vi "통신.vi"(8 "error in":errorcluster) -> (0 "error out":errorcluster, 3 "Boolean":bool)   [LabVIEW 2023]
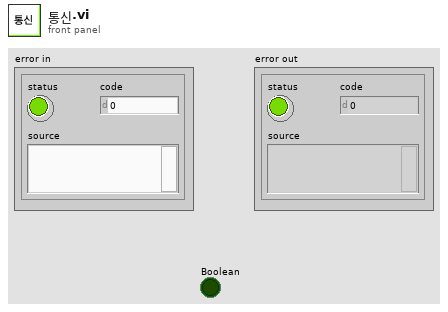
[diagram p1: front panel]
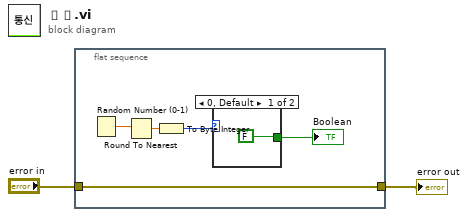
[diagram p0: block diagram]
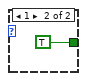
[diagram p2: hidden frame]
diagram:
  n1 = flat-sequence {
    tunnel: "error in" -> [w3]
    tunnel: [w3] -> w1
    frame #0 {
      n2 = Random Number (0-1)() -> (number: 0 to 1=w7:dbl)
      n3 = Round To Nearest(number=w7) -> (nearest integer value=w6:dbl)
      n4 = To Byte Integer(number=w6) -> (8bit integer=w5:i8)
      n5 = case shown="0, Default" w5 {
        tunnel: [FALSE TRUE] -> w4
        frame 0, Default {
        }
        frame 1 {
        }
      }
      "Boolean" <- w4
    }
  }
  "error out" <- w1
